vi "CheckVISAtype.vi"(11 "VISA Refnum in":refnum<visa-resource-name>) -> (2 "size":i32, 3 "data string":string)   [LabVIEW 2016]
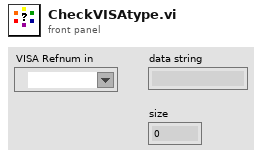
[diagram p1: front panel]
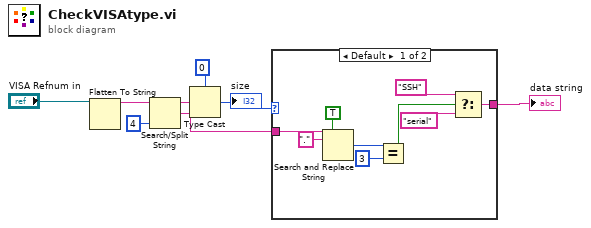
[diagram p0: block diagram]
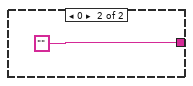
[diagram p2: hidden frame]
diagram:
  n1 = Flatten To String(anything="VISA Refnum in") -> (data string=w4:string)  [unwired: 3 in, 2 out]
  n2 = Search/Split String(string=w4, offset (0)=4) -> (substring before match=w6:string, match + rest of string=w1:string)  [unwired: 1 in, 1 out]
  n3 = Type Cast(type=0 ("offset (0)"), x=w6) -> (*(type *) &x=w3:i32)
  "size" <- w3
  n4 = case shown="Default" w3 {
    tunnel: [w9 ""] -> w2
    tunnel: w1 -> [w17 _]
    frame Default {
      n5 = Search and Replace String(replace all?=TRUE ("replace all? (F)"), input string=w17, search string=".") -> (number of replacements=w14:i32)  [unwired: 5 in, 3 out]
      n6 = Equal?(x=w14, y=3) -> (x = y?=w12:bool)
      n7 = Select(t="SSH" ("search string"), s=w12, f="serial" ("search string")) -> (s? t:f=w9:string)
    }
    frame 0 {
    }
  }
  "data string" <- w2
